vi "Cleanup.vi"(8 "error in (no error)":errorcluster, 11 "StringStream in":refnum<class "StringStream.lvclass">) -> (0 "error out":errorcluster, 3 "StringStream out":refnum<class "StringStream.lvclass">)   [LabVIEW 2020, in "IO.lvlib" / "StringStream.lvclass"]
uses:
  StringStream.lvclass
  StringStream.lvclass/StringStream.ctl
  Stream/Stream.lvclass
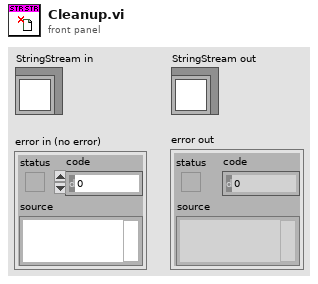
[diagram p1: front panel]
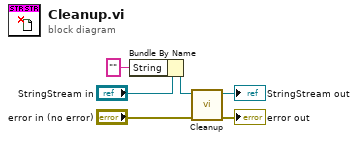
[diagram p0: block diagram]
diagram:
  n1 = Bundle By Name(cluster="StringStream in", "String"="") -> (w4:refnum<class "StringStream.lvclass">)
  n2 = call-parent "Cleanup.vi"("error in (no error)"="error in (no error)", "Stream in"=w4) -> ("error out"=→"error out":errorcluster, "Stream out"=→"StringStream out":refnum<class "StringStream.lvclass">)  [unwired: 8 in]
